vi "_UserDialog Choose Filename.vi"(0 "VI Default Path":path, 7 "Default file name":string, 11 "error in (no error)":errorcluster, 13 "Not In <help> directory? (Yes: T)":bool=TRUE) -> (4 "HTML File Path":path, 6 "Images Folder Path":path, 8 "LV <help> directory path":path, 14 "Cancelled by User?":bool, 15 "error out":errorcluster)   [LabVIEW 2012]
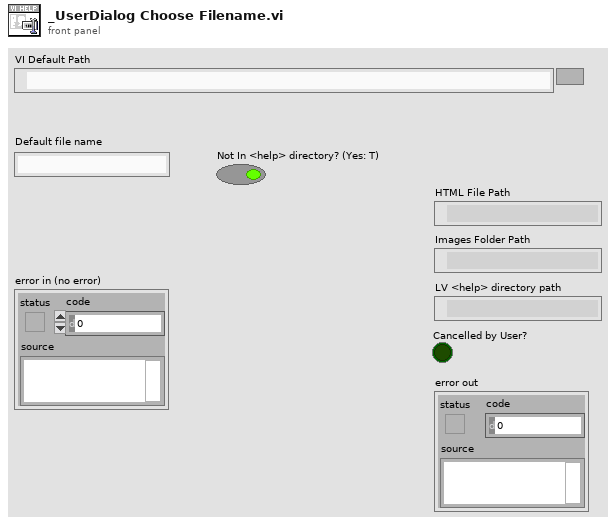
[diagram p1: front panel]
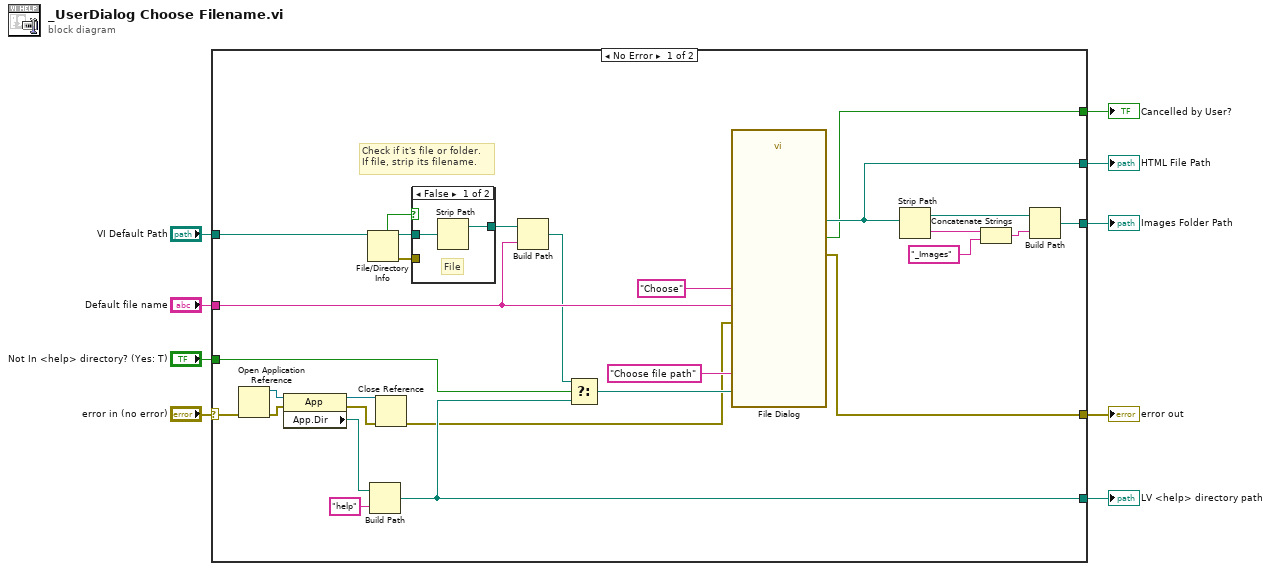
[diagram p0: block diagram]
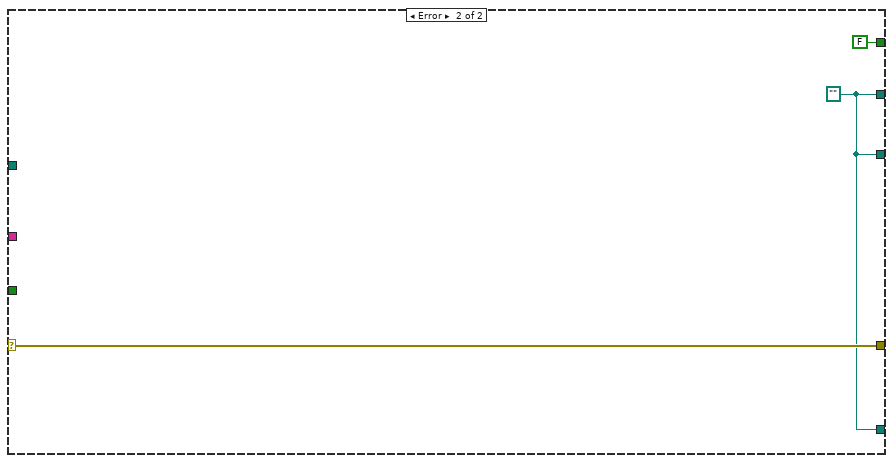
[diagram p3: hidden frame]
diagram:
  n1 = case shown="No Error" "error in (no error)" {
    selector: "error in (no error)" -> [w10 w43]
    tunnel: [w37 w41] -> w9
    tunnel: [w36 w41] -> w8
    tunnel: "Default file name" -> [w34 _]
    tunnel: "Not In <help> directory? (Yes: T)" -> [w30 _]
    tunnel: [w23 w41] -> w5
    tunnel: [w16 w43] -> w4
    tunnel: [w15 FALSE ("cancelled")] -> w3
    tunnel: "VI Default Path" -> [w14 _]
    frame No Error {
      # "Check if it's file or folder.\nIf file, strip its filename."
      n2 = Open Application Reference(8:w10) -> (0:w25:errorcluster, 3:w24:refnum<vi>)  [unwired: 3 in]
      n3 = property class="App"(reference=w24, error in=w25) -> (reference out=w26:refnum<vi>, error out=w27:errorcluster, "App.Dir"=w28:path)
      n4 = File/Directory Info(path=w14) -> (path out=w13:path, directory=w12:bool, error out=w11:errorcluster)  [unwired: 1 in, 4 out]
      n5 = Build Path(base path=w28, name or relative path="help") -> (appended path=w23:path)
      n6 = Close Reference(reference=w26, error in (no error)=w27) -> (error out=w17:errorcluster)
      n7 = case shown="False" w12 {
        tunnel: [w39 w40] -> w22
        tunnel: w13 -> [w38 w40]
        tunnel: w11 -> [_ _]
        frame False {
          # "File"
          n8 = Strip Path(path=w38) -> (stripped path=w39:path)  [unwired: 1 out]
        }
        frame True {
          # "Directory"
        }
      }
      n9 = Build Path(base path=w22, name or relative path=w34) -> (appended path=w20:path)
      n10 = Select(t=w20, s=w30, f=w23) -> (s? t:f=w19:path)
      n11 = call "File Dialog"("start path"=w19, "prompt"="Choose file path", "button label"="Choose", "default name"=w34, "error in"=w17) -> ("selected path"=w36:path, "cancelled"=w15:bool, "error out"=w16:errorcluster)  [unwired: 7 in, 1 out]
      n12 = Strip Path(path=w36) -> (stripped path=w35:path, name=w32:string)
      n13 = Concatenate Strings(w32, "_Images" ("name or relative path")) -> (w31:string)
      n14 = Build Path(base path=w35, name or relative path=w31) -> (appended path=w37:path)
    }
    frame Error {
      w41 = path ""
    }
  }
  "error out" <- w4
  "HTML File Path" <- w8
  "Images Folder Path" <- w9
  "LV <help> directory path" <- w5
  "Cancelled by User?" <- w3
